vi "Determine_Save_Order.vi"(8 "error in (no error)":errorcluster, 10 "all VIs in memory":string[](array[string]), 11 "AB_Source_Library in":refnum<class "AB_Source_Library.lvclass">) -> (0 "error out":errorcluster, 2 "saveOrder":i32, 3 "AB_Source_Library out":refnum<class "AB_Source_Library.lvclass">)   [LabVIEW 2020, in "AB_Source_Library.lvclass"]
uses:
  <vilib>/AppBuilder/AB_Classes/Source/Library/AB_Source_Library.lvclass
  e:/builds/penguin/labview/branches/2020/dev/dist/vi.lib/AppBuilder/AB_Classes/Source/AB_Source.lvclass
  <vilib>/AppBuilder/AB_Classes/Source/AB_Source.lvclass
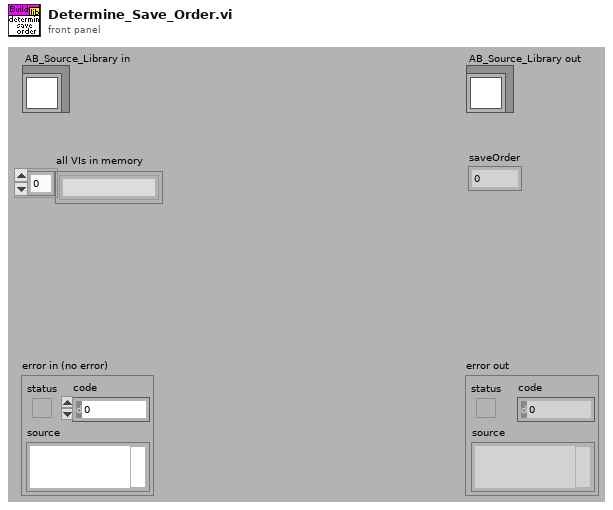
[diagram p1: front panel]
types:
  T1 = typedef "AB_Source.ctl" = cluster{"path":path, "itemID":string, "parentIndex":i32, "sourceInclusion":T2, "destinationIndex":i32, "properties":T3[], "newName":string, "lvfile":bool, "valid":bool, "eng_inBuild":bool, "eng_isNonVILink":bool, "Amalgamation":bool, "Amalgamation Piece":bool, "eng_delimitedName":string, "preventRename":bool}
  T2 = typedef "AB_Source_Inclusion.ctl" = enum16{"IncludeIfReferenced", "Include", "Exclude", "TopLevel"}
  T3 = typedef "AB_Source_Properties.ctl" = cluster{"sourcePropertyType":T4, "value":variant}
  T4 = typedef "AB_Source_Property_Type.ctl" = enum16{"Remove block diagram", "Remove front panel", "Password", "Window has title bar", "Show menu bar", "Show vertical scroll bar", "Show horizontal scroll bar", "Show toolbar", "Show Abort button", "Show fp when called", "Window behavior", "Allow user to close window", "Window run-time position", "Run when opened", "Allow debugging", "Auto error handling", "Generate guard code", "Use stack variables", "Expression folding", "Integer only", "Inline subVI"}
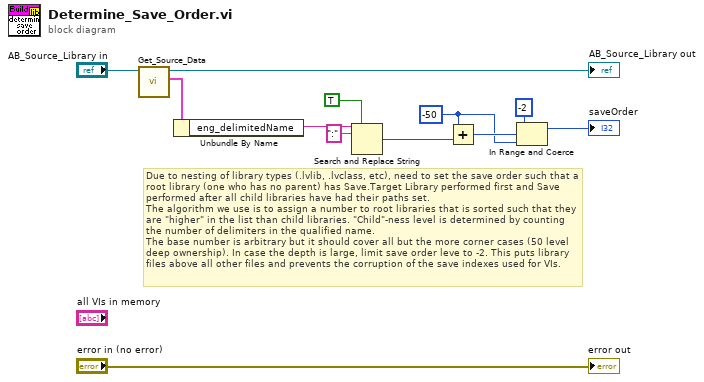
[diagram p0: block diagram]
diagram:
  w5 = -50 ("saveOrder")
  # "Due to nesting of library types (.lvlib, .lvclass, etc), need to set the save order such that a root library (one who has no parent) has Save.Target Library performed first and Save performed after all child libraries have had their paths set. \nThe algorithm we use is to assign a number to root libraries that is sorted such that they are \"higher\" in the list than child libraries. \"Child\"-ness level is determined by counting the number of delimiters in the qualified name. \nThe base number is arbitrary but it should cover all but the more corner cases (50 level deep ownership). In case the depth is large, limit save order leve to -2. This puts library files above all other files and prevents the corruption of the save indexes used for VIs."
  n1 = call <vilib>:"Get_Source_Data.vi"("Class in"="AB_Source_Library in") -> ("data"=w1:T1, "Class out"=→"AB_Source_Library out":refnum<class "AB_Source_Library.lvclass">)  [unwired: 8 in, 1 out]
  n2 = Unbundle By Name(w1) -> ("eng_delimitedName"=w11:string)
  n3 = Search and Replace String(replace all?=TRUE ("replace all? (F)"), input string=w11, search string=":") -> (number of replacements=w8:i32)  [unwired: 5 in, 3 out]
  n4 = Add(x=w5, y=w8) -> (x+y=w6:i32)
  n5 = In Range and Coerce(upper limit=-2 ("x"), x=w6, lower limit=w5) -> (coerced(x)=→"saveOrder":i32)  [unwired: 1 out]
  "error out" <- "error in (no error)"
